vi "Read_Cluster_Values_Benchmark.vi"() -> ()   [LabVIEW 2018]
uses:
  NiFpga.dll
panel:
  out "Waveform Graph":dbl[](graph)
  out "Average":dbl
  out "U8":u32
  out "i16":i16
  out "error code":i32
  out "FXP":dbl
  out "error out":errorcluster
  in  "Error In":errorcluster
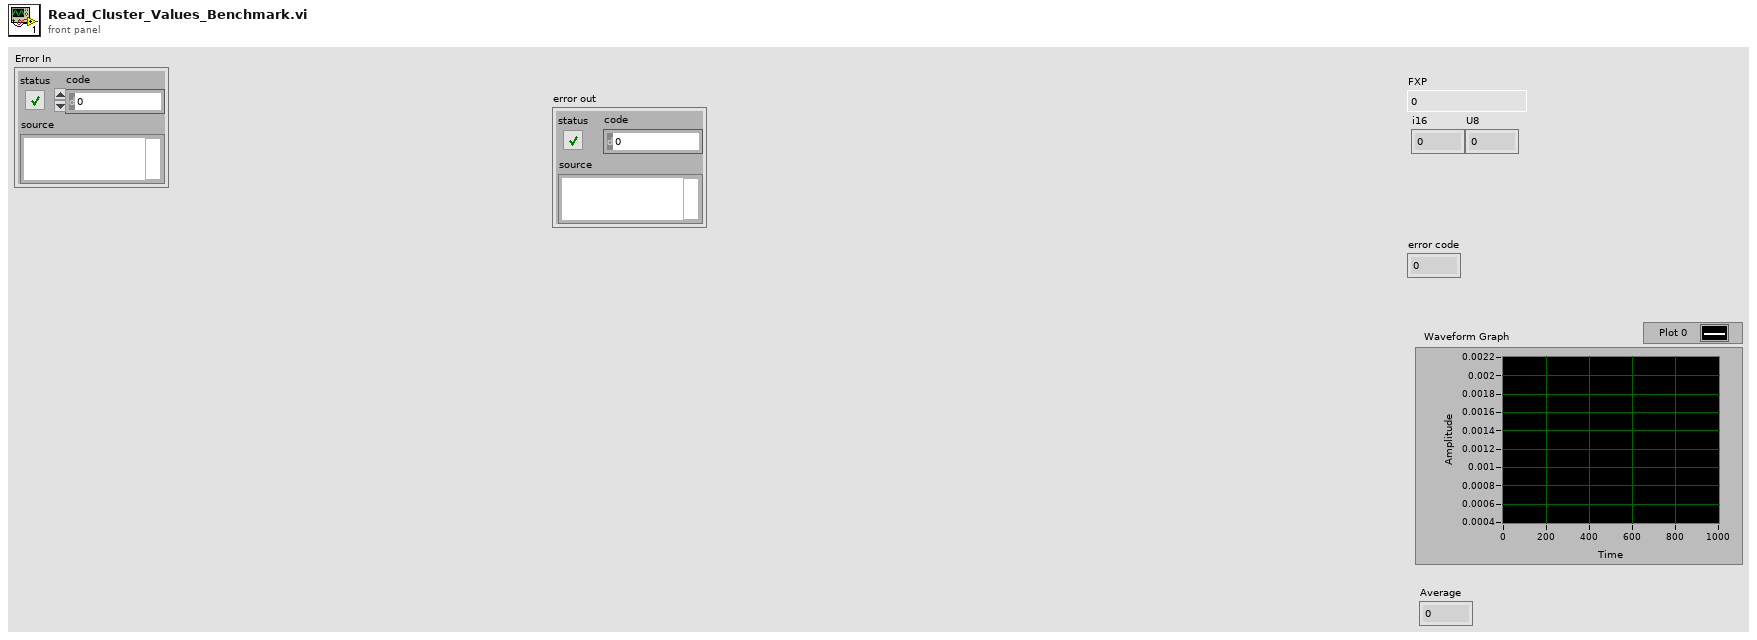
[diagram p1: front panel]
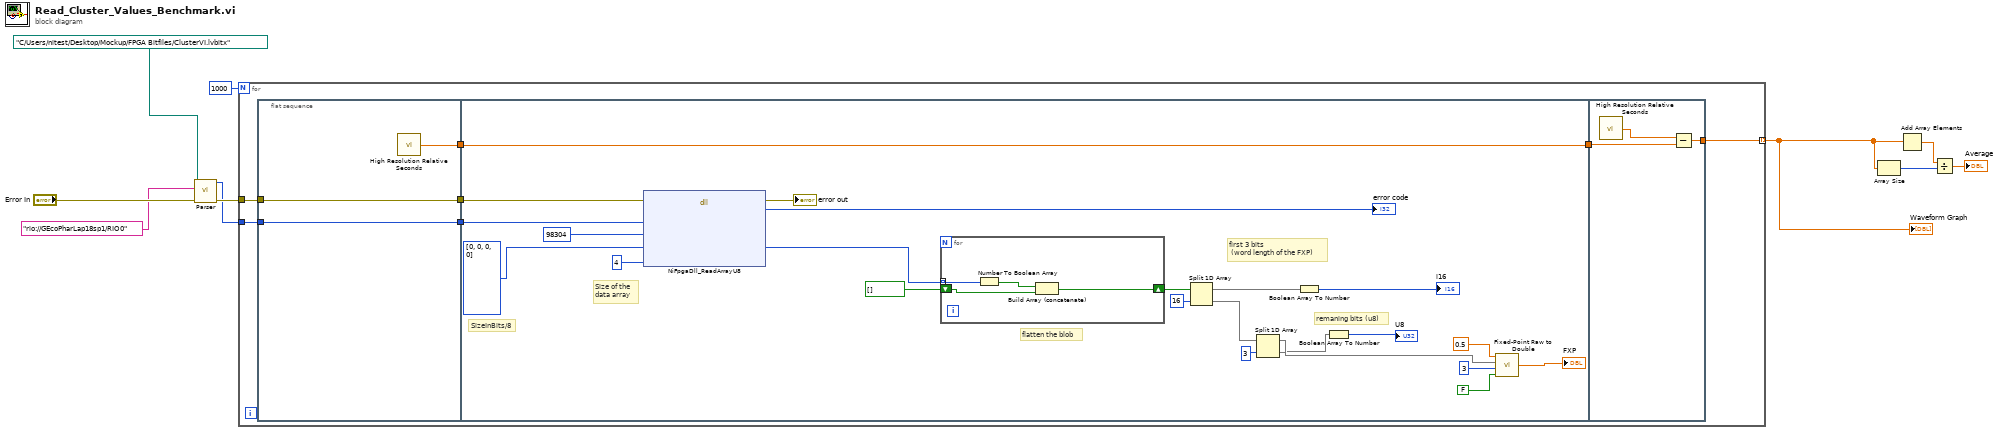
[diagram p0: block diagram]
diagram:
  n1 = call "Parser.vi"("error in (no error)"="Error In", "RIO device address"="rio://GEcoPharLap18sp1/RIO0" ("Device address"), "bitfile path"=path "C:/Users/nitest/Desktop/Mockup/FPGA Bitfiles/ClusterVI.lvbitx" ("Bitfile path")) -> ("error out"=w8:errorcluster, "session out"=w6:u64)  [unwired: 6 in, 1 out]
  n2 = for {
    N: 1000 -> [_]
    tunnel: w8 -> [w17]
    tunnel: w6 -> [w16]
    tunnel: [w11] -> w1 mode=indexing
    n3 = flat-sequence {
      tunnel: w16 -> [w19]
      tunnel: w17 -> [w20]
      tunnel: [w20] -> w15
      tunnel: [w19] -> w14
      tunnel: [w18] -> w13
      tunnel: w15 -> [w42]
      tunnel: w14 -> [w41]
      tunnel: w13 -> [w21]
      tunnel: [w21] -> w12
      tunnel: w12 -> [w49]
      tunnel: [w48] -> w11
      frame #0 {
        n4 = call <vilib>:"High Resolution Relative Seconds.vi"() -> ("relative seconds"=w18:dbl)
      }
      frame #1 {
        # "remaning bits (u8)"
        # "first 3 bits\n (word length of the FXP)"
        # "flatten the blob"
        # "Size of the \ndata array"
        # "SizeInBits/8"
        n5 = dll-call lib="NiFpga.*" fn="NiFpgaDll_ReadArrayU8"(error in=w42, "session"=w41, "offset"=u32 98304, "data"=u8[] [0, 0, 0, 0], "count"=u8 4) -> (error out=→"error out":errorcluster, "status"=→"error code":i32, "data"=w37:u8[])  [unwired: 5 in, 1 out]
        n6 = for {
          shift-right: [w45] -> w31
          shift-left: bool[] [] ("element") -> [w46]
          tunnel: w37 -> [w44] mode=indexing
          n7 = Number To Boolean Array(number=w44) -> (Boolean array=w47:bool[])
          n8 = Build Array (concatenate)(w47, w46) -> (w45:bool[])
        }
        n9 = Split 1D Array(array=w31, index=16) -> (first subarray=w26:bool[], second subarray=w28:bool[])
        n10 = Split 1D Array(array=w28, index=3) -> (first subarray=w23:bool[], second subarray=w22:bool[])
        n11 = Boolean Array To Number(Boolean array=w26) -> (number=→"i16":u32)
        n12 = Boolean Array To Number(Boolean array=w22) -> (number=→"U8":u32)
        n13 = call "Fixed-Point Raw to Double.vi"("Signed?"=FALSE, "Word Length"=u8 3, "Data"=w23, "Delta"=0.5) -> ("value"=→"FXP":dbl)
      }
      frame #2 {
        n14 = call <vilib>:"High Resolution Relative Seconds.vi"() -> ("relative seconds"=w50:dbl)
        n15 = Subtract(x=w50, y=w49) -> (x-y=w48:dbl)
      }
    }
  }
  "Waveform Graph" <- w1
  n16 = Array Size(array=w1) -> (size(s)=w3:i32)
  n17 = Add Array Elements(numeric array=w1) -> (sum=w4:dbl)
  n18 = Divide(x=w4, y=w3) -> (x/y=→"Average":dbl)
